vi "control.vi"() -> ()   [LabVIEW 2020]
uses:
  G_Pulsador_Stop_Sistema.vi
  G_Pulsador_Reset_Sistema.vi
  G_Pulsador_Star_Puesto_1.vi
  G_Pulsador_Start_Puesto_2.vi
  G_Posicion_Inicial_Cilindro_5.vi
  G_Posicion_Final_Cilindro_5.vi
  G_Posicion_Inicial_Cilindro_4.vi
  G_Posicion_Final_Cilindro_4.vi
  G_Posicion_Inicial_Cilindro_1.vi
  G_Posicion_Final_Cilindro_1.vi
  G_Posicion_Final_Cilindro_3.vi
  G_Posicion_Inicial_Cilindro_3.vi
  G_Posicion_Inicial_Cilindro_2.vi
  G_Posicion_Final_Cilindro_2.vi
  G_Indicador_Atras_Cilindro_2.vi
  G_Indicador_Adelante_Cilindro_2.vi
  G_Indicador_Atras_Cilindro_4.vi
  G_Indicador_Adelante_Cilindro_4.vi
  G_Indicador_Atras_Pegamento.vi
  G_Indicador_Adelante_Pegamento.vi
  G_Indicador_Adelante_Cilindro_5.vi
  G_Indicador_Atras_Cilindro_5.vi
  G_Indicador_Adelante_Cilindro_3.vi
  G_Indicador_Atras_Cilindro_3.vi
panel:
  in  "pause":bool
  in  "paro":bool
  in  "start p1 2":bool
  in  "start  p2":bool
  out "acaba ciclo p2":bool
  out "acaba ciclo p1":bool
  in  "stop":bool
  in  "stop 2":bool
  # "stop"
  # "pause"
  # "p1"
  # "p2"
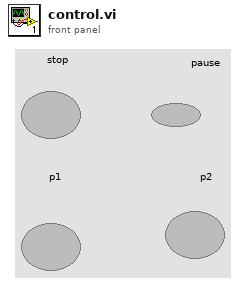
[diagram p1: front panel]
types:
  T1 = enum16{"reposo", "avance p1", "subir pega 1", "retoceso 1", "subir p 2", "estado inicial"}
  T2 = enum16{"reposo", "avance 1", "subir pega 1", "retroceso 1", "subir p1", "espera segundos", "estado inicial", ""}
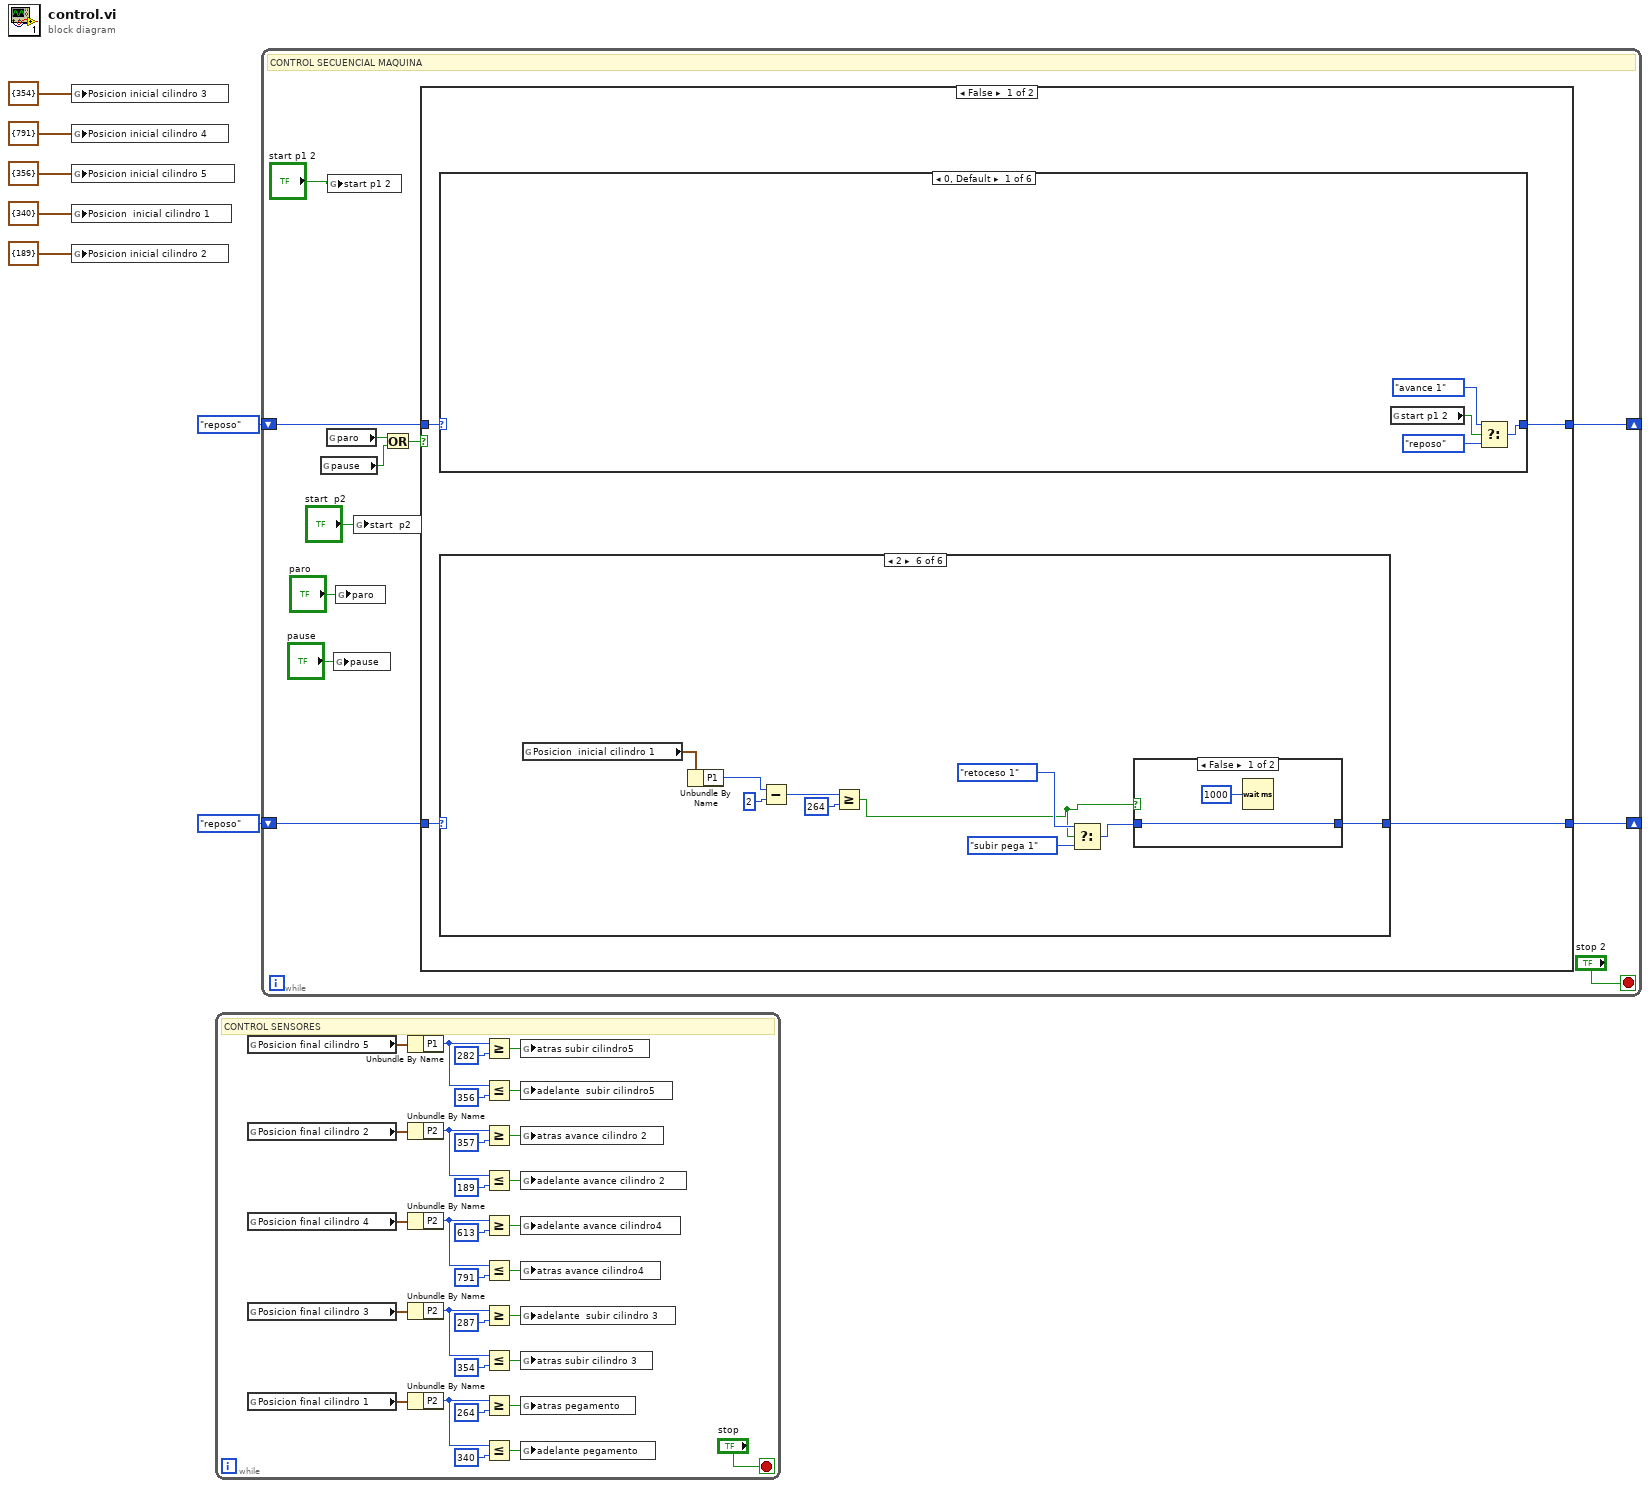
[diagram p0: block diagram]
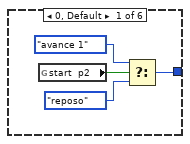
[diagram p2: hidden frame]
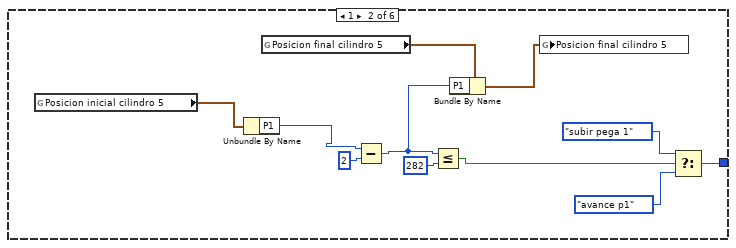
[diagram p3: hidden frame]
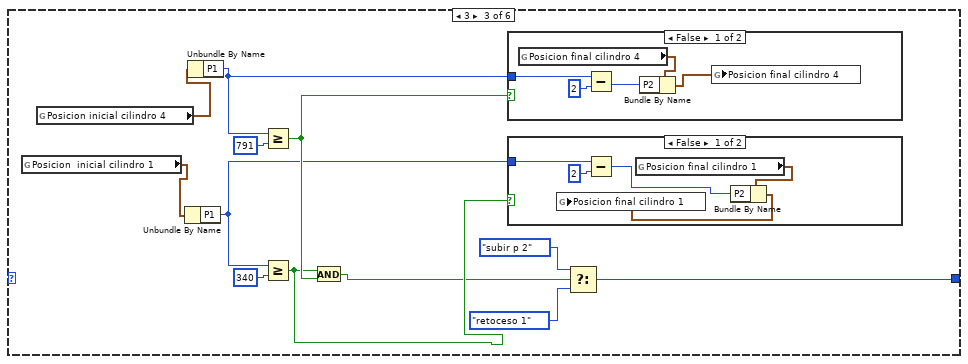
[diagram p4: hidden frame]
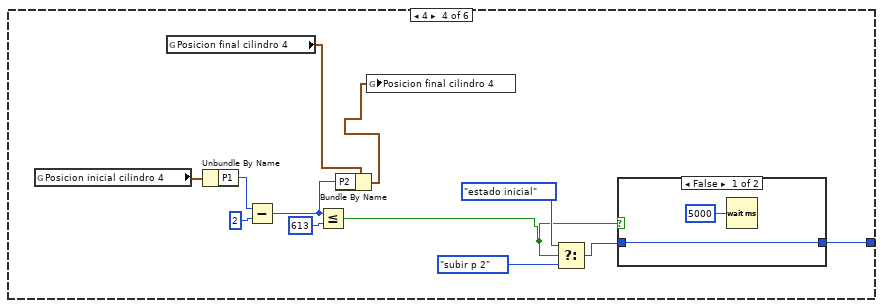
[diagram p7: hidden frame]
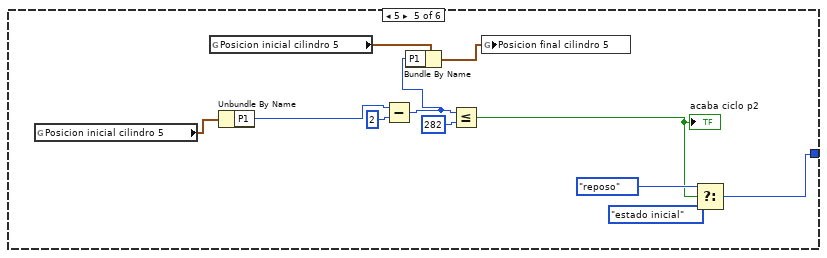
[diagram p9: hidden frame]
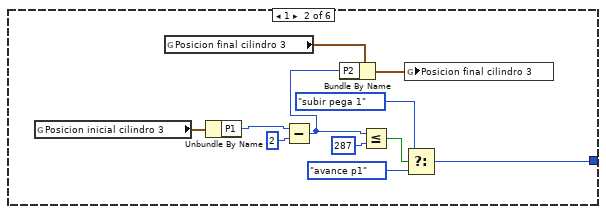
[diagram p11: hidden frame]
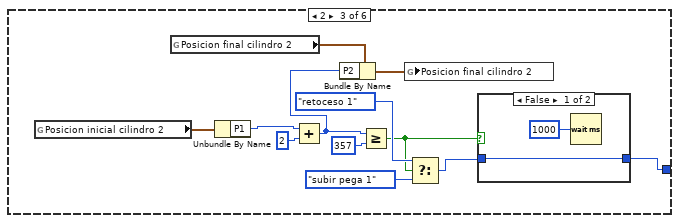
[diagram p12: hidden frame]
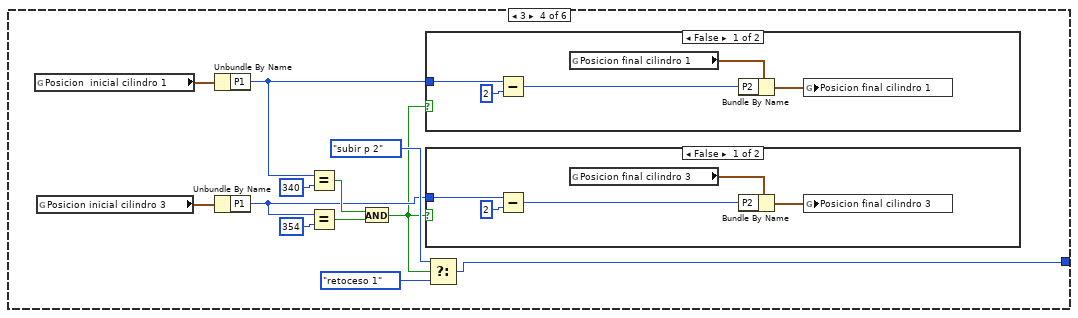
[diagram p14: hidden frame]
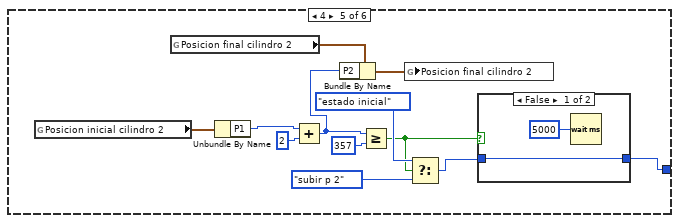
[diagram p17: hidden frame]
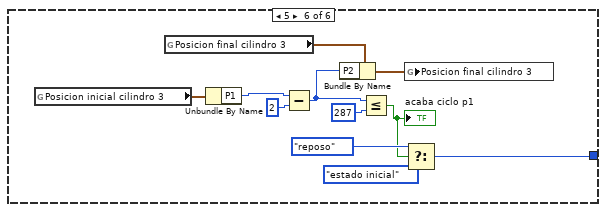
[diagram p19: hidden frame]
diagram:
  n1 = global write "G_Posicion_Inicial_Cilindro_3.vi" "Posicion inicial cilindro 3"(cluster{"P1":i32} {"P1"=354} ("Posicion inicial cilindro 3")) -> ()
  n2 = global write "G_Posicion_Inicial_Cilindro_4.vi" "Posicion inicial cilindro 4"(cluster{"P1":i32} {"P1"=791} ("Posicion inicial cilindro 4")) -> ()
  n3 = global write "G_Posicion_Inicial_Cilindro_5.vi" "Posicion inicial cilindro 5"(cluster{"P1":i32} {"P1"=356} ("Posicion inicial cilindro 5")) -> ()
  n4 = global write "G_Posicion_Inicial_Cilindro_1.vi" "Posicion  inicial cilindro 1"(cluster{"P1":i32} {"P1"=340} ("Posicion  inicial cilindro 1")) -> ()
  n5 = global write "G_Posicion_Inicial_Cilindro_2.vi" "Posicion inicial cilindro 2"(cluster{"P1":i32} {"P1"=189} ("Posicion inicial cilindro 2")) -> ()
  n6 = while {
    stop <- "stop" stop-if-true
    # "CONTROL SENSORES"
    n7 = global read "G_Posicion_Final_Cilindro_5.vi" "Posicion final cilindro 5"() -> (w15:cluster{"P1":i32})
    n8 = global read "G_Posicion_Final_Cilindro_2.vi" "Posicion final cilindro 2"() -> (w27:cluster{"P2":i32})
    n9 = global read "G_Posicion_Final_Cilindro_4.vi" "Posicion final cilindro 4"() -> (w23:cluster{"P2":i32})
    n10 = global read "G_Posicion_Final_Cilindro_3.vi" "Posicion final cilindro 3"() -> (w11:cluster{"P2":i32})
    n11 = global read "G_Posicion_Final_Cilindro_1.vi" "Posicion final cilindro 1"() -> (w19:cluster{"P2":i32})
    n12 = Unbundle By Name(w15) -> ("P1"=w14:i32)
    n13 = Unbundle By Name(w27) -> ("P2"=w26:i32)
    n14 = Unbundle By Name(w23) -> ("P2"=w22:i32)
    n15 = Unbundle By Name(w11) -> ("P2"=w10:i32)
    n16 = Unbundle By Name(w19) -> ("P2"=w18:i32)
    n17 = Greater Or Equal?(x=w14, y=282) -> (x >= y?=w12:bool)
    n18 = Less Or Equal?(x=w14, y=356) -> (x <= y?=w13:bool)
    n19 = Greater Or Equal?(x=w26, y=357) -> (x >= y?=w24:bool)
    n20 = Less Or Equal?(x=w26, y=189) -> (x <= y?=w25:bool)
    n21 = Greater Or Equal?(x=w22, y=613) -> (x >= y?=w21:bool)
    n22 = Less Or Equal?(x=w22, y=791) -> (x <= y?=w20:bool)
    n23 = Greater Or Equal?(x=w10, y=287) -> (x >= y?=w9:bool)
    n24 = Less Or Equal?(x=w10, y=354) -> (x <= y?=w8:bool)
    n25 = Greater Or Equal?(x=w18, y=264) -> (x >= y?=w16:bool)
    n26 = Less Or Equal?(x=w18, y=340) -> (x <= y?=w17:bool)
    n27 = global write "G_Indicador_Atras_Cilindro_5.vi" "atras subir cilindro5"(w12) -> ()
    n28 = global write "G_Indicador_Adelante_Cilindro_5.vi" "adelante  subir cilindro5"(w13) -> ()
    n29 = global write "G_Indicador_Atras_Cilindro_2.vi" "atras avance cilindro 2"(w24) -> ()
    n30 = global write "G_Indicador_Adelante_Cilindro_2.vi" "adelante avance cilindro 2"(w25) -> ()
    n31 = global write "G_Indicador_Adelante_Cilindro_4.vi" "adelante avance cilindro4"(w21) -> ()
    n32 = global write "G_Indicador_Atras_Cilindro_4.vi" "atras avance cilindro4"(w20) -> ()
    n33 = global write "G_Indicador_Adelante_Cilindro_3.vi" "adelante  subir cilindro 3"(w9) -> ()
    n34 = global write "G_Indicador_Atras_Cilindro_3.vi" "atras subir cilindro 3"(w8) -> ()
    n35 = global write "G_Indicador_Atras_Pegamento.vi" "atras pegamento"(w16) -> ()
    n36 = global write "G_Indicador_Adelante_Pegamento.vi" "adelante pegamento"(w17) -> ()
  }
  n37 = while {
    shift-right: [w49] -> _
    shift-left: T1."reposo" -> [w50]
    shift-right: [w47] -> _
    shift-left: T1."reposo" -> [w48]
    stop <- "stop 2" stop-if-true
    # "CONTROL SECUENCIAL MAQUINA"
    n38 = global read "G_Pulsador_Reset_Sistema.vi" "pause"() -> (w43:bool)
    n39 = global read "G_Pulsador_Stop_Sistema.vi" "paro"() -> (w44:bool)
    n40 = global write "G_Pulsador_Star_Puesto_1.vi" "start p1 2"("start p1 2") -> ()
    n41 = global write "G_Pulsador_Reset_Sistema.vi" "pause"("pause") -> ()
    n42 = global write "G_Pulsador_Stop_Sistema.vi" "paro"("paro") -> ()
    n43 = global write "G_Pulsador_Start_Puesto_2.vi" "start  p2"("start  p2") -> ()
    n44 = Or(x=w44, y=w43) -> (x .or. y?=w45:bool)
    n45 = case shown="False" w45 {
      tunnel: w50 -> [w51 w209]
      tunnel: [w53 w209] -> w49
      tunnel: w48 -> [w54 w210]
      tunnel: [w52 w210] -> w47
      frame False {
        n46 = case shown="0, Default" w51 {
          tunnel: [w132 w142 w152 w166 w189 w204] -> w53
          frame 0, Default {
            n47 = global read "G_Pulsador_Star_Puesto_1.vi" "start p1 2"() -> (w131:bool)
            n48 = Select(t=T2."avance 1", s=w131, f=T2."reposo") -> (s? t:f=w132:T2)
          }
          frame 1 {
            n49 = global read "G_Posicion_Inicial_Cilindro_3.vi" "Posicion inicial cilindro 3"() -> (w140:cluster{"P1":i32})
            n50 = global read "G_Posicion_Final_Cilindro_3.vi" "Posicion final cilindro 3"() -> (w137:cluster{"P2":i32})
            n51 = Unbundle By Name(w140) -> ("P1"=w139:i32)
            n52 = Subtract(x=w139, y=2) -> (x-y=w135:i32)
            n53 = Bundle By Name(cluster=w137, "P2"=w135) -> (w136:cluster{"P2":i32})
            n54 = Less Or Equal?(x=w135, y=287) -> (x <= y?=w138:bool)
            n55 = global write "G_Posicion_Final_Cilindro_3.vi" "Posicion final cilindro 3"(w136) -> ()
            n56 = Select(t=T1."subir pega 1", s=w138, f=T1."avance p1") -> (s? t:f=w142:T1)
          }
          frame 2 {
            n57 = global read "G_Posicion_Inicial_Cilindro_2.vi" "Posicion inicial cilindro 2"() -> (w151:cluster{"P1":i32})
            n58 = global read "G_Posicion_Final_Cilindro_2.vi" "Posicion final cilindro 2"() -> (w147:cluster{"P2":i32})
            n59 = Unbundle By Name(w151) -> ("P1"=w150:i32)
            n60 = Add(x=w150, y=2) -> (x+y=w148:i32)
            n61 = Bundle By Name(cluster=w147, "P2"=w148) -> (w146:cluster{"P2":i32})
            n62 = Greater Or Equal?(x=w148, y=357) -> (x >= y?=w149:bool)
            n63 = global write "G_Posicion_Final_Cilindro_2.vi" "Posicion final cilindro 2"(w146) -> ()
            n64 = Select(t=T1."retoceso 1", s=w149, f=T1."subir pega 1") -> (s? t:f=w153:T1)
            n65 = case shown="False" w149 {
              tunnel: w153 -> [w158 w160]
              tunnel: [w158 w160] -> w152
              frame False {
                n66 = Wait (ms)(milliseconds to wait=u32 1000) -> ()  [unwired: 1 out]
              }
              frame True {
              }
            }
          }
          frame 3 {
            n67 = global read "G_Posicion_Inicial_Cilindro_1.vi" "Posicion  inicial cilindro 1"() -> (w165:cluster{"P1":i32})
            n68 = global read "G_Posicion_Inicial_Cilindro_3.vi" "Posicion inicial cilindro 3"() -> (w163:cluster{"P1":i32})
            n69 = Unbundle By Name(w165) -> ("P1"=w164:i32)
            n70 = Unbundle By Name(w163) -> ("P1"=w162:i32)
            n71 = Equal?(x=w164, y=340) -> (x = y?=w168:bool)
            n72 = Equal?(x=w162, y=354) -> (x = y?=w167:bool)
            n73 = And(x=w168, y=w167) -> (x .and. y?=w161:bool)
            n74 = case shown="False" w161 {
              tunnel: w164 -> [w176 _]
              frame False {
                n75 = Subtract(x=w176, y=2) -> (x-y=w175:i32)
                n76 = global read "G_Posicion_Final_Cilindro_1.vi" "Posicion final cilindro 1"() -> (w174:cluster{"P2":i32})
                n77 = Bundle By Name(cluster=w174, "P2"=w175) -> (w173:cluster{"P2":i32})
                n78 = global write "G_Posicion_Final_Cilindro_1.vi" "Posicion final cilindro 1"(w173) -> ()
              }
              frame True {
              }
            }
            n79 = case shown="False" w161 {
              tunnel: w162 -> [w181 _]
              frame False {
                n80 = Subtract(x=w181, y=2) -> (x-y=w180:i32)
                n81 = global read "G_Posicion_Final_Cilindro_3.vi" "Posicion final cilindro 3"() -> (w178:cluster{"P2":i32})
                n82 = Bundle By Name(cluster=w178, "P2"=w180) -> (w179:cluster{"P2":i32})
                n83 = global write "G_Posicion_Final_Cilindro_3.vi" "Posicion final cilindro 3"(w179) -> ()
              }
              frame True {
              }
            }
            n84 = Select(t=T1."subir p 2", s=w161, f=T1."retoceso 1") -> (s? t:f=w166:T1)
          }
          frame 4 {
            n85 = global read "G_Posicion_Inicial_Cilindro_2.vi" "Posicion inicial cilindro 2"() -> (w188:cluster{"P1":i32})
            n86 = global read "G_Posicion_Final_Cilindro_2.vi" "Posicion final cilindro 2"() -> (w183:cluster{"P2":i32})
            n87 = Unbundle By Name(w188) -> ("P1"=w187:i32)
            n88 = Add(x=w187, y=2) -> (x+y=w185:i32)
            n89 = Bundle By Name(cluster=w183, "P2"=w185) -> (w184:cluster{"P2":i32})
            n90 = Greater Or Equal?(x=w185, y=357) -> (x >= y?=w186:bool)
            n91 = global write "G_Posicion_Final_Cilindro_2.vi" "Posicion final cilindro 2"(w184) -> ()
            n92 = Select(t=T1."estado inicial", s=w186, f=T1."subir p 2") -> (s? t:f=w190:T1)
            n93 = case shown="False" w186 {
              tunnel: w190 -> [w196 w197]
              tunnel: [w196 w197] -> w189
              frame False {
                n94 = Wait (ms)(milliseconds to wait=u32 5000) -> ()  [unwired: 1 out]
              }
              frame True {
              }
            }
          }
          frame 5 {
            n95 = global read "G_Posicion_Inicial_Cilindro_3.vi" "Posicion inicial cilindro 3"() -> (w203:cluster{"P1":i32})
            n96 = global read "G_Posicion_Final_Cilindro_3.vi" "Posicion final cilindro 3"() -> (w198:cluster{"P2":i32})
            n97 = Unbundle By Name(w203) -> ("P1"=w202:i32)
            n98 = Subtract(x=w202, y=2) -> (x-y=w200:i32)
            n99 = Bundle By Name(cluster=w198, "P2"=w200) -> (w199:cluster{"P2":i32})
            n100 = Less Or Equal?(x=w200, y=287) -> (x <= y?=w201:bool)
            "acaba ciclo p1" <- w201
            n101 = global write "G_Posicion_Final_Cilindro_3.vi" "Posicion final cilindro 3"(w199) -> ()
            n102 = Select(t=T1."reposo", s=w201, f=T1."estado inicial") -> (s? t:f=w204:T1)
          }
        }
        n103 = case shown="2" w54 {
          tunnel: [w56 w65 w77 w98 w113 w121] -> w52
          frame 0, Default {
            n104 = global read "G_Pulsador_Start_Puesto_2.vi" "start  p2"() -> (w55:bool)
            n105 = Select(t=T2."avance 1", s=w55, f=T2."reposo") -> (s? t:f=w56:T2)
          }
          frame 1 {
            n106 = global read "G_Posicion_Inicial_Cilindro_5.vi" "Posicion inicial cilindro 5"() -> (w64:cluster{"P1":i32})
            n107 = Unbundle By Name(w64) -> ("P1"=w63:i32)
            n108 = global read "G_Posicion_Final_Cilindro_5.vi" "Posicion final cilindro 5"() -> (w61:cluster{"P1":i32})
            n109 = Subtract(x=w63, y=2) -> (x-y=w62:i32)
            n110 = Less Or Equal?(x=w62, y=282) -> (x <= y?=w59:bool)
            n111 = Bundle By Name(cluster=w61, "P1"=w62) -> (w60:cluster{"P1":i32})
            n112 = global write "G_Posicion_Final_Cilindro_5.vi" "Posicion final cilindro 5"(w60) -> ()
            n113 = Select(t=T1."subir pega 1", s=w59, f=T1."avance p1") -> (s? t:f=w65:T1)
          }
          frame 3 {
            n114 = global read "G_Posicion_Inicial_Cilindro_1.vi" "Posicion  inicial cilindro 1"() -> (w73:cluster{"P1":i32})
            n115 = global read "G_Posicion_Inicial_Cilindro_4.vi" "Posicion inicial cilindro 4"() -> (w76:cluster{"P1":i32})
            n116 = Unbundle By Name(w73) -> ("P1"=w72:i32)
            n117 = Unbundle By Name(w76) -> ("P1"=w75:i32)
            n118 = Greater Or Equal?(x=w75, y=791) -> (x >= y?=w74:bool)
            n119 = Greater Or Equal?(x=w72, y=340) -> (x >= y?=w71:bool)
            n120 = And(x=w71, y=w74) -> (x .and. y?=w70:bool)
            n121 = case shown="False" w74 {
              tunnel: w75 -> [w91 _]
              frame False {
                n122 = global read "G_Posicion_Final_Cilindro_4.vi" "Posicion final cilindro 4"() -> (w88:cluster{"P2":i32})
                n123 = Subtract(x=w91, y=2) -> (x-y=w89:i32)
                n124 = Bundle By Name(cluster=w88, "P2"=w89) -> (w87:cluster{"P2":i32})
                n125 = global write "G_Posicion_Final_Cilindro_4.vi" "Posicion final cilindro 4"(w87) -> ()
              }
              frame True {
              }
            }
            n126 = case shown="False" w71 {
              tunnel: w72 -> [w85 _]
              frame False {
                n127 = Subtract(x=w85, y=2) -> (x-y=w84:i32)
                n128 = global read "G_Posicion_Final_Cilindro_1.vi" "Posicion final cilindro 1"() -> (w83:cluster{"P2":i32})
                n129 = Bundle By Name(cluster=w83, "P2"=w84) -> (w82:cluster{"P2":i32})
                n130 = global write "G_Posicion_Final_Cilindro_1.vi" "Posicion final cilindro 1"(w82) -> ()
              }
              frame True {
              }
            }
            n131 = Select(t=T1."subir p 2", s=w70, f=T1."retoceso 1") -> (s? t:f=w77:T1)
          }
          frame 4 {
            n132 = global read "G_Posicion_Inicial_Cilindro_4.vi" "Posicion inicial cilindro 4"() -> (w97:cluster{"P1":i32})
            n133 = global read "G_Posicion_Final_Cilindro_4.vi" "Posicion final cilindro 4"() -> (w92:cluster{"P2":i32})
            n134 = Unbundle By Name(w97) -> ("P1"=w96:i32)
            n135 = Subtract(x=w96, y=2) -> (x-y=w94:i32)
            n136 = Less Or Equal?(x=w94, y=613) -> (x <= y?=w95:bool)
            n137 = Bundle By Name(cluster=w92, "P2"=w94) -> (w93:cluster{"P2":i32})
            n138 = global write "G_Posicion_Final_Cilindro_4.vi" "Posicion final cilindro 4"(w93) -> ()
            n139 = Select(t=T1."estado inicial", s=w95, f=T1."subir p 2") -> (s? t:f=w103:T1)
            n140 = case shown="False" w95 {
              tunnel: w103 -> [w105 w106]
              tunnel: [w105 w106] -> w98
              frame False {
                n141 = Wait (ms)(milliseconds to wait=u32 5000) -> ()  [unwired: 1 out]
              }
              frame True {
              }
            }
          }
          frame 5 {
            n142 = global read "G_Posicion_Inicial_Cilindro_5.vi" "Posicion inicial cilindro 5"() -> (w112:cluster{"P1":i32})
            n143 = global read "G_Posicion_Inicial_Cilindro_5.vi" "Posicion inicial cilindro 5"() -> (w107:cluster{"P1":i32})
            n144 = Unbundle By Name(w112) -> ("P1"=w111:i32)
            n145 = Subtract(x=w111, y=2) -> (x-y=w109:i32)
            n146 = Bundle By Name(cluster=w107, "P1"=w109) -> (w108:cluster{"P1":i32})
            n147 = Less Or Equal?(x=w109, y=282) -> (x <= y?=w110:bool)
            "acaba ciclo p2" <- w110
            n148 = global write "G_Posicion_Final_Cilindro_5.vi" "Posicion final cilindro 5"(w108) -> ()
            n149 = Select(t=T1."reposo", s=w110, f=T1."estado inicial") -> (s? t:f=w113:T1)
          }
          frame 2 {
            n150 = global read "G_Posicion_Inicial_Cilindro_1.vi" "Posicion  inicial cilindro 1"() -> (w120:cluster{"P1":i32})
            n151 = Unbundle By Name(w120) -> ("P1"=w119:i32)
            n152 = Subtract(x=w119, y=2) -> (x-y=w123:i32)
            n153 = Greater Or Equal?(x=w123, y=264) -> (x >= y?=w118:bool)
            n154 = Select(t=T1."retoceso 1", s=w118, f=T1."subir pega 1") -> (s? t:f=w127:T1)
            n155 = case shown="False" w118 {
              tunnel: w127 -> [w128 w130]
              tunnel: [w128 w130] -> w121
              frame False {
                n156 = Wait (ms)(milliseconds to wait=u32 1000) -> ()  [unwired: 1 out]
              }
              frame True {
              }
            }
          }
        }
      }
      frame True {
      }
    }
  }
